vi "niFpga wdp fft DIT 8spc.vi"(0 "real data in":fxp<+/-,8,1>[](array[numeric])=[0.0, 0.0, 0.0, 0.0, 0.0, 0.0, 0.0, 0.0], 5 "imaginary data in":fxp<+/-,8,1>[](array[numeric])=[0.0, 0.0, 0.0, 0.0, 0.0, 0.0, 0.0, 0.0], 9 "input frame start":bool, 12 "enable":bool) -> (3 "data indices":u16[](array[numeric]), 4 "real data out":fxp<+,8,1>[](array[numeric]), 6 "imaginary data out":fxp<+,8,1>[](array[numeric]), 10 "output valid":bool, 14 "ready for frame":bool, 15 "output frame start":bool)   [LabVIEW 2017]
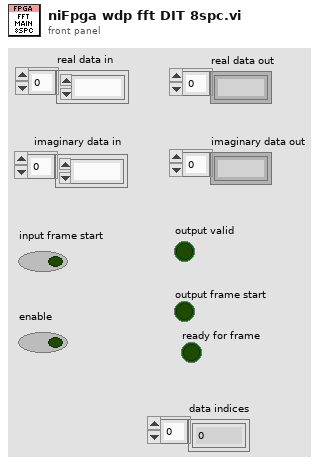
[diagram p1: front panel]
types:
  T1 = cluster{"internal input type":fxp<+/-,8,1>, "internal input type":fxp<+/-,8,1>}
  T2 = cluster{"twiddle factor type":fxp<+/-,16,2>, "twiddle factor type":fxp<+/-,16,2>}[]
  T3 = cluster{"x-y":fxp<+/-,19,12>, "x-y":fxp<+/-,19,12>}
  T4 = cluster{"x+y":fxp<+/-,19,12>, "x+y":fxp<+/-,19,12>}
  T5 = cluster{"x+y":fxp<+/-,19,12>, "x+y":fxp<+/-,19,12>}[]
  T6 = cluster{"x-y":fxp<+/-,19,12>, "x-y":fxp<+/-,19,12>}[]
  T7 = cluster{"data re":fxp<+/-,8,1>, "data im":fxp<+/-,8,1>}[]
  T8 = cluster{"x-y":fxp<+/-,20,13>, "x-y":fxp<+/-,20,13>}[]
  T9 = cluster{"x-y":fxp<+/-,20,13>, "x-y":fxp<+/-,20,13>}
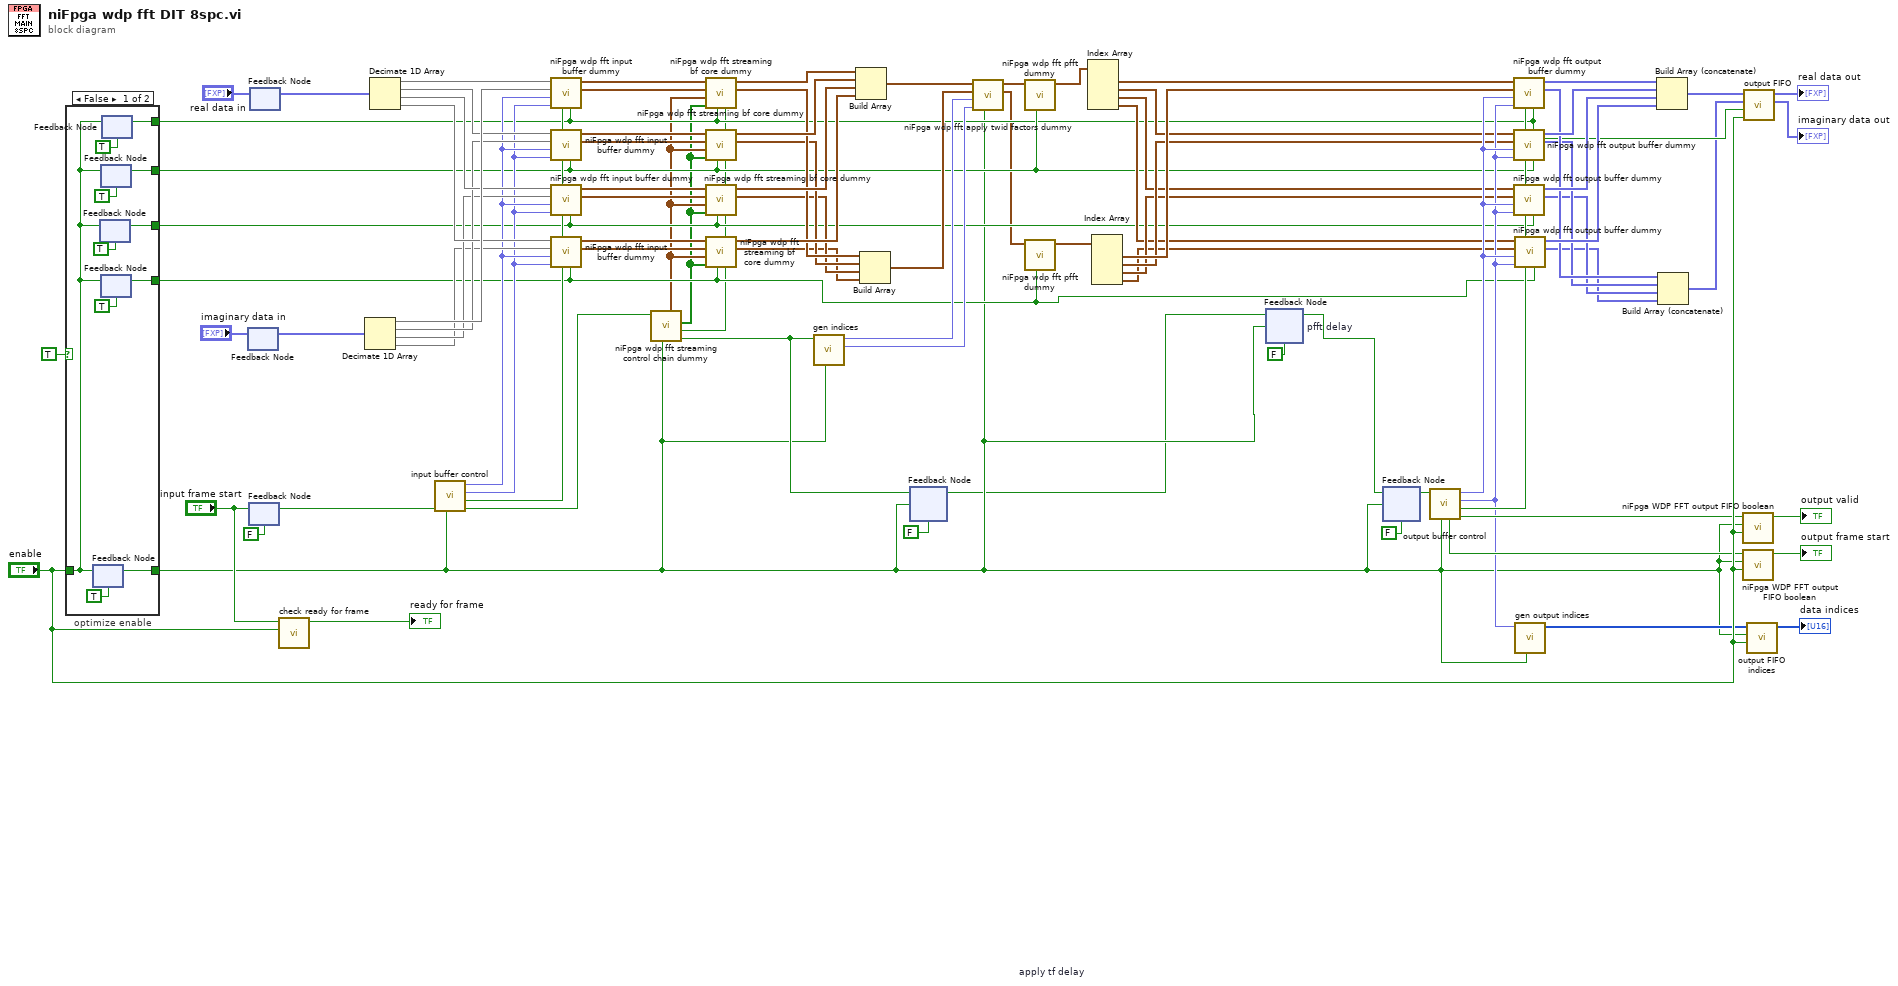
[diagram p0: block diagram]
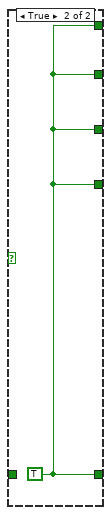
[diagram p2: hidden frame]
diagram:
  n1 = case "optimize enable" shown="False" TRUE {
    tunnel: [w101 w102] -> w16
    tunnel: [w100 w102] -> w15
    tunnel: [w99 w102] -> w14
    tunnel: [w98 w102] -> w13
    tunnel: "enable" -> [w97 _]
    tunnel: [w96 w102] -> w8
    frame False {
      n2 = feedback #1(TRUE ("enable")) -> (w96:bool)
      n3 = feedback-in #1(w97) -> ()
      n4 = feedback #2(TRUE ("enable")) -> (w100:bool)
      n5 = feedback-in #2(w97) -> ()
      n6 = feedback #3(TRUE ("enable")) -> (w101:bool)
      n7 = feedback-in #3(w97) -> ()
      n8 = feedback #4(TRUE ("enable")) -> (w99:bool)
      n9 = feedback-in #4(w97) -> ()
      n10 = feedback #5(TRUE ("enable")) -> (w98:bool)
      n11 = feedback-in #5(w97) -> ()
    }
    frame True {
      w102 = TRUE
    }
  }
  n12 = feedback #6() -> (w60:fxp<+/-,8,1>[])  [unwired: 1 in]
  n13 = feedback-in #6("imaginary data in") -> ()
  n14 = feedback #7(FALSE ("enable")) -> (w83:bool)
  n15 = feedback-in #7("input frame start") -> ()
  n16 = feedback #8() -> (w62:fxp<+/-,8,1>[])  [unwired: 1 in]
  n17 = feedback-in #8("real data in") -> ()
  n18 = call "check ready for frame"("enable"="enable", "frame start in"="input frame start") -> ("ready for frame"=→"ready for frame":bool)  [unwired: 9 in]
  n19 = Decimate 1D Array(w60) -> (w59:fxp<+/-,8,1>[], w49:fxp<+/-,8,1>[], w48:fxp<+/-,8,1>[], w47:fxp<+/-,8,1>[])
  n20 = Decimate 1D Array(w62) -> (w61:fxp<+/-,8,1>[], w58:fxp<+/-,8,1>[], w51:fxp<+/-,8,1>[], w50:fxp<+/-,8,1>[])
  n21 = call "input buffer control"("enable"=w8, "frame start in"=w83) -> ("frame start out"=w26:bool, "write memory 2?"=w40:bool, "read index"=w45:fxp<+,9,9>, "write index"=w46:fxp<+,8,8>)  [unwired: 6 in]
  n22 = call <vilib>:"niFpga wdp fft input buffer dummy.vi"("enable"=w13, "write memory 2?"=w40, "read index"=w45, "write index"=w46, "data in im"=w59, "data in re"=w61) -> ("data out 1"=w63:T1, "data out 0"=w64:T1)  [unwired: 4 in]
  n23 = call <vilib>:"niFpga wdp fft input buffer dummy.vi"("enable"=w16, "write memory 2?"=w40, "read index"=w45, "write index"=w46, "data in im"=w49, "data in re"=w58) -> ("data out 1"=w56:T1, "data out 0"=w57:T1)  [unwired: 4 in]
  n24 = call <vilib>:"niFpga wdp fft input buffer dummy.vi"("enable"=w15, "write memory 2?"=w40, "read index"=w45, "write index"=w46, "data in im"=w48, "data in re"=w51) -> ("data out 1"=w54:T1, "data out 0"=w55:T1)  [unwired: 4 in]
  n25 = call <vilib>:"niFpga wdp fft input buffer dummy.vi"("enable"=w14, "write memory 2?"=w40, "read index"=w45, "write index"=w46, "data in im"=w47, "data in re"=w50) -> ("data out 1"=w52:T1, "data out 0"=w53:T1)  [unwired: 4 in]
  n26 = call <vilib>:"niFpga wdp fft streaming control chain dummy.vi"("enable"=w8, "input frame start"=w26) -> ("frame start"=w25:bool, "index=0?"=w5:bool, "switch"=w4:bool[], "twiddle factors"=w6:T2)  [unwired: 5 in, 1 out]
  n27 = call <vilib>:"niFpga wdp fft streaming bf core dummy.vi"("index=0?"=w5, "enable"=w13, "switch"=w4, "twiddle factors"=w6, "data in 1"=w63, "data in 0"=w64) -> ("data out 1"=w78:T3, "data out 0"=w82:T4)  [unwired: 4 in]
  n28 = call <vilib>:"niFpga wdp fft streaming bf core dummy.vi"("index=0?"=w5, "enable"=w16, "switch"=w4, "twiddle factors"=w6, "data in 1"=w56, "data in 0"=w57) -> ("data out 1"=w77:T3, "data out 0"=w81:T4)  [unwired: 4 in]
  n29 = call <vilib>:"niFpga wdp fft streaming bf core dummy.vi"("index=0?"=w5, "enable"=w15, "switch"=w4, "twiddle factors"=w6, "data in 1"=w54, "data in 0"=w55) -> ("data out 1"=w76:T3, "data out 0"=w80:T4)  [unwired: 4 in]
  n30 = call <vilib>:"niFpga wdp fft streaming bf core dummy.vi"("index=0?"=w5, "enable"=w14, "switch"=w4, "twiddle factors"=w6, "data in 1"=w52, "data in 0"=w53) -> ("data out 1"=w75:T3, "data out 0"=w79:T4)  [unwired: 4 in]
  n31 = call "gen indices"("enable"=w8, "frame start"=w25) -> ("data index 1"=w28:fxp<+,10,10>, "data index 0"=w29:fxp<+,10,10>)  [unwired: 8 in]
  n32 = Build Array(w82, w81, w80, w79) -> (w74:T5)
  n33 = Build Array(w78, w77, w76, w75) -> (w73:T6)
  n34 = feedback #9 "apply tf delay"(FALSE) -> (w7:bool)
  n35 = feedback-in #9(w25, w8) -> ()
  n36 = call <vilib>:"niFpga wdp fft apply twid factors dummy.vi"("enable"=w8, "data index 1"=w28, "data index 0"=w29, "data in 1"=w73, "data in 0"=w74) -> ("data out 1"=w2:T7, "data out 0"=w3:T7)  [unwired: 5 in]
  n37 = call <vilib>:"niFpga wdp fft pfft dummy.vi"("enable"=w16, "data in"=w3) -> ("data out"=w90:T8)  [unwired: 9 in]
  n38 = call <vilib>:"niFpga wdp fft pfft dummy.vi"("enable"=w14, "data in"=w2) -> ("data out"=w89:T8)  [unwired: 9 in]
  n39 = Index Array(array=w90) -> (element #1=w24:T9, element #2=w22:T9, element #3=w20:T9, element #4=w18:T9)  [unwired: 4 in]
  n40 = Index Array(array=w89) -> (element #1=w23:T9, element #2=w21:T9, element #3=w19:T9, element #4=w17:T9)  [unwired: 4 in]
  n41 = feedback #10 "pfft delay"(FALSE) -> (w11:bool)
  n42 = feedback-in #10(w7, w8) -> ()
  n43 = feedback #11 ("delay")(FALSE) -> (w10:bool)
  n44 = feedback-in #11(w11, w8) -> ()
  n45 = call "output buffer control"("enable"=w8, "frame start"=w10) -> ("output valid?"=w36:bool, "memory switch"=w33:bool, "read index"=w32:fxp<+,4,4>, "write index"=w34:fxp<+,9,9>, "frame start?"=w35:bool)  [unwired: 5 in]
  n46 = call <vilib>:"niFpga wdp fft output buffer dummy.vi"("enable"=w13, "memory switch"=w33, "read index"=w32, "write index"=w34, "data in 1"=w23, "data in 0"=w24) -> ("data out im"=w68:fxp<+/-,32,16>[], "data out re"=w72:fxp<+/-,32,16>[])  [unwired: 4 in]
  n47 = call <vilib>:"niFpga wdp fft output buffer dummy.vi"("enable"=w16, "memory switch"=w33, "read index"=w32, "write index"=w34, "data in 1"=w21, "data in 0"=w22) -> ("data out im"=w67:fxp<+/-,32,16>[], "data out re"=w71:fxp<+/-,32,16>[])  [unwired: 4 in]
  n48 = call <vilib>:"niFpga wdp fft output buffer dummy.vi"("enable"=w15, "memory switch"=w33, "read index"=w32, "write index"=w34, "data in 1"=w19, "data in 0"=w20) -> ("data out im"=w66:fxp<+/-,32,16>[], "data out re"=w70:fxp<+/-,32,16>[])  [unwired: 4 in]
  n49 = call <vilib>:"niFpga wdp fft output buffer dummy.vi"("enable"=w14, "memory switch"=w33, "read index"=w32, "write index"=w34, "data in 1"=w17, "data in 0"=w18) -> ("data out im"=w65:fxp<+/-,32,16>[], "data out re"=w69:fxp<+/-,32,16>[])  [unwired: 4 in]
  n50 = call "gen output indices"("enable"=w8, "index"=w32) -> ("data indices"=w31:u16[])  [unwired: 9 in]
  n51 = Build Array (concatenate)(w72, w71, w70, w69) -> (w43:fxp<+/-,32,16>[])
  n52 = Build Array (concatenate)(w68, w67, w66, w65) -> (w9:fxp<+/-,32,16>[])
  n53 = call <vilib>:"niFpga WDP FFT output FIFO boolean.vi"("enable"="enable", "enable with delay"=w8, "boolean in"=w36) -> ("boolean out"=→"output valid":bool)  [unwired: 8 in]
  n54 = call <vilib>:"niFpga WDP FFT output FIFO boolean.vi"("enable"="enable", "enable with delay"=w8, "boolean in"=w35) -> ("boolean out"=→"output frame start":bool)  [unwired: 8 in]
  n55 = call "output FIFO"("enable"="enable", "enable with delay"=w13, "data in 1"=w9, "data in 0"=w43) -> ("data out 1"=→"imaginary data out":fxp<+,8,1>[], "data out 0"=→"real data out":fxp<+,8,1>[])  [unwired: 6 in]
  n56 = call "output FIFO indices"("enable"="enable", "enable with delay"=w8, "data in"=w31) -> ("data out"=→"data indices":u16[])  [unwired: 8 in]
